vi "Arduino com - VISA Serial.vi"() -> ()   [LabVIEW 2024]
uses:
  <vilib>/Instr/_visa.llb/VISA Configure Serial Port (Instr).vi
panel:
  in  "Boolean":bool
  in  "VISA resource name":refnum<visa-resource-name>
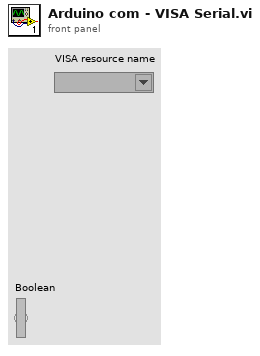
[diagram p1: front panel]
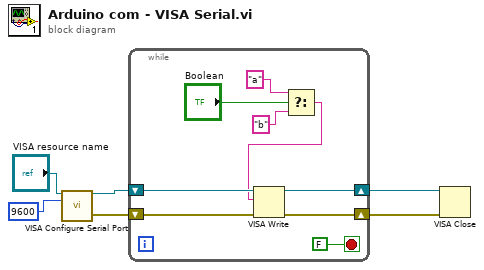
[diagram p0: block diagram]
diagram:
  n1 = call-poly "VISA Configure Serial Port"("VISA resource name"="VISA resource name", "baud rate (9600)"=u32 9600) -> ("VISA resource name out"=w6:refnum<visa-resource-name>, "error out"=w3:errorcluster)  [unwired: 12 in]
  n2 = while {
    shift-right: [w14] -> w5
    shift-left: w6 -> [w15]
    shift-right: [w13] -> w4
    shift-left: w3 -> [w12]
    stop <- FALSE stop-if-true
    n3 = Select(t="a", s="Boolean", f="b") -> (s? t:f=w9:string)
    n4 = VISA Write(VISA resource name=w15, write buffer=w9, error in (no error)=w12) -> (VISA resource name out=w14:refnum<visa-resource-name>, error out=w13:errorcluster)  [unwired: 1 out]
  }
  n5 = VISA Close(VISA resource name=w5, error in (no error)=w4) -> ()  [unwired: 1 out]
